vi "turning.vi"(10 "Turn time":dbl, 11 "clock anticlock":string) -> (3 "angle moved":dbl)   [LabVIEW 2015]
panel:
  out "finish angle":dbl
  out "Start angle":dbl
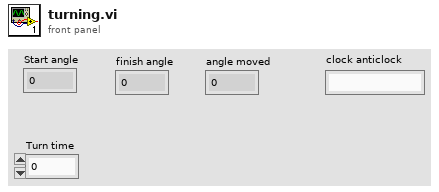
[diagram p1: front panel]
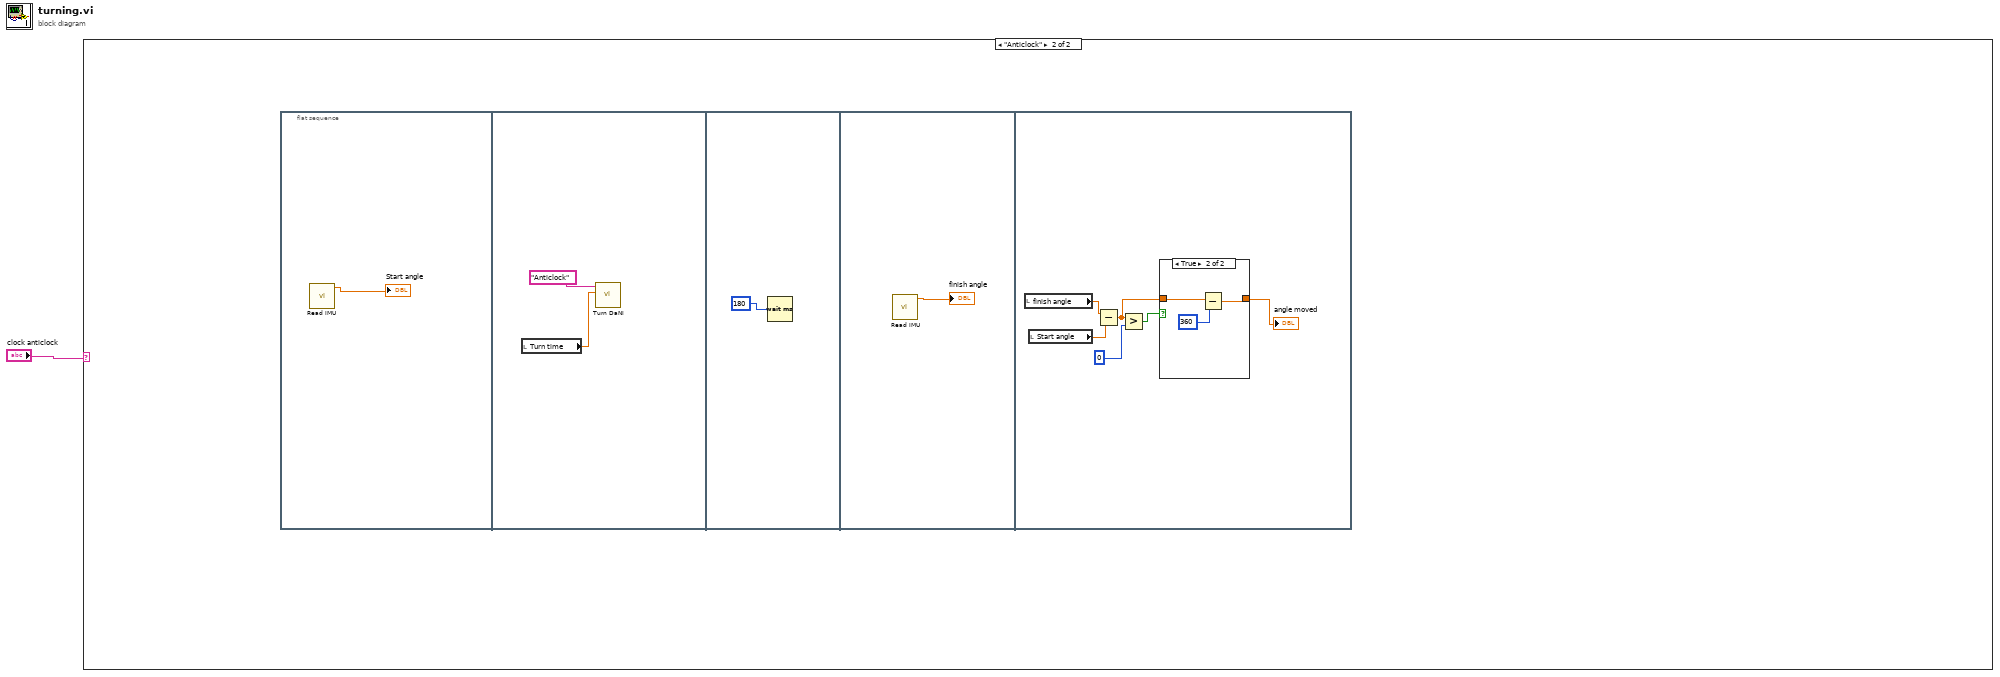
[diagram p0: block diagram]
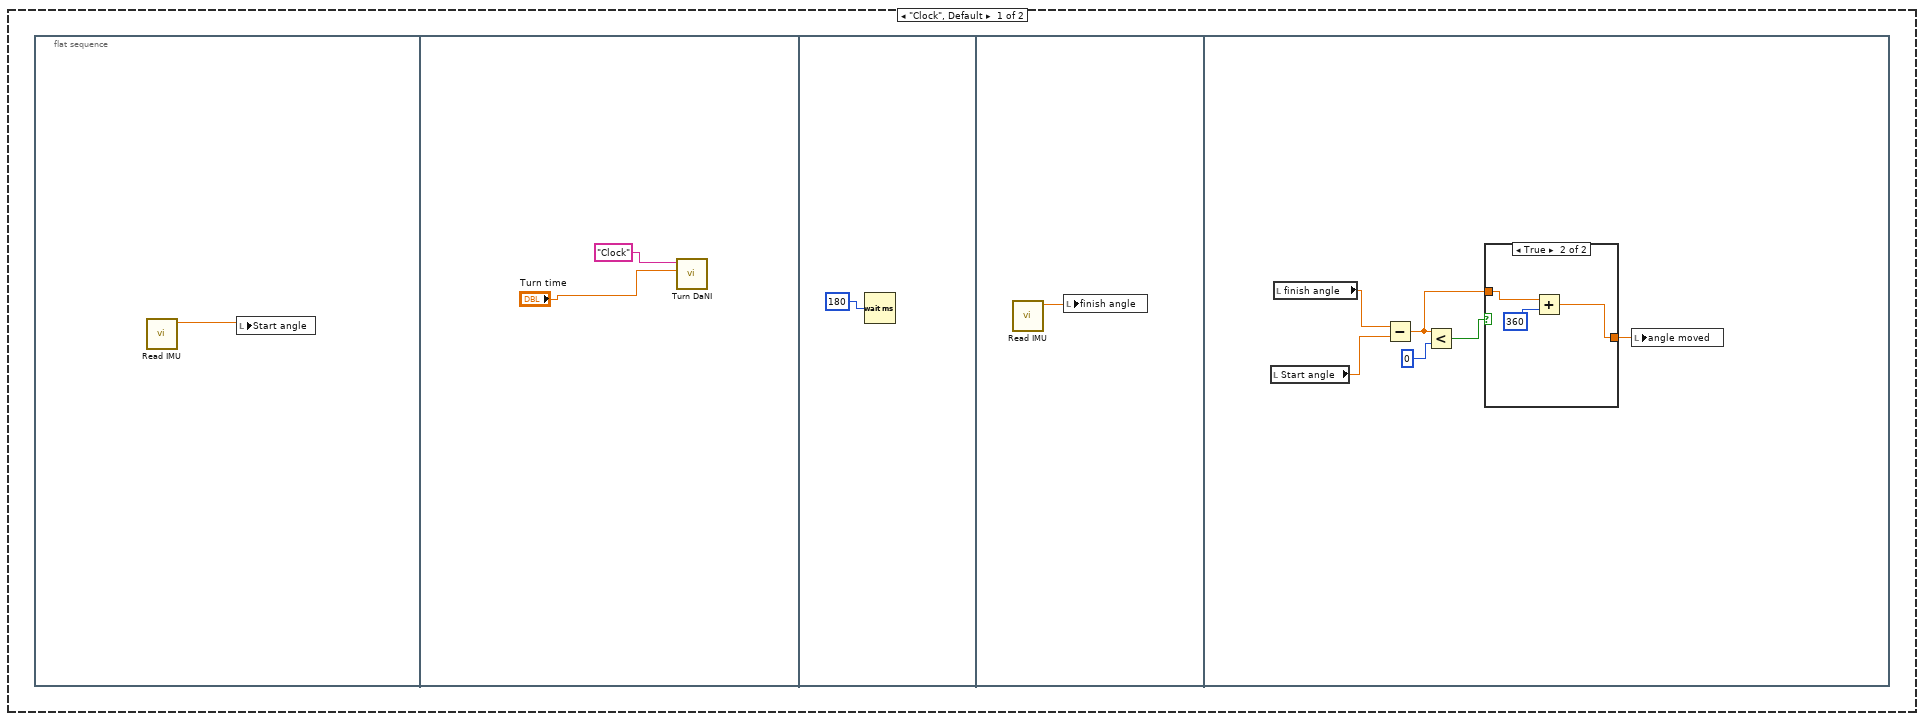
[diagram p2: hidden frame]
diagram:
  n1 = case shown="\"Anticlock\"" "clock anticlock" {
    frame "Clock", Default {
      n2 = flat-sequence {
        frame #0 {
          n3 = call "Read IMU.vi"() -> ("Output Angle"=w2:dbl)  [unwired: 10 in, 1 out]
          n4 = local write "Start angle"(w2) -> ()
        }
        frame #1 {
          n5 = call "Turn DaNI.vi"("wait time (ms)"="Turn time", "Clockwise/Anticlocwise"="Clock") -> ()  [unwired: 10 in]
        }
        frame #2 {
          n6 = Wait (ms)(milliseconds to wait=180) -> ()  [unwired: 1 out]
        }
        frame #3 {
          n7 = call "Read IMU.vi"() -> ("Output Angle"=w6:dbl)  [unwired: 10 in, 1 out]
          n8 = local write "finish angle"(w6) -> ()
        }
        frame #4 {
          n9 = local read "Start angle"() -> (w12:dbl)
          n10 = local read "finish angle"() -> (w11:dbl)
          n11 = Subtract(x=w11, y=w12) -> (x-y=w8:dbl)
          n12 = Less?(x=w8, y=0) -> (x < y?=w9:bool)
          n13 = case shown="True" w9 {
            tunnel: w8 -> [w13 w16]
            tunnel: [w13 w14] -> w7
            frame False {
            }
            frame True {
              n14 = Add(x=w16, y=360) -> (x+y=w14:dbl)
            }
          }
          n15 = local write "angle moved"(w7) -> ()
        }
      }
    }
    frame "Anticlock" {
      n16 = flat-sequence {
        frame #0 {
          n17 = call "Read IMU.vi"() -> ("Output Angle"=→"Start angle":dbl)  [unwired: 10 in, 1 out]
        }
        frame #1 {
          n18 = local read "Turn time"() -> (w18:dbl)
          n19 = call "Turn DaNI.vi"("wait time (ms)"=w18, "Clockwise/Anticlocwise"="Anticlock") -> ()  [unwired: 10 in]
        }
        frame #2 {
          n20 = Wait (ms)(milliseconds to wait=180) -> ()  [unwired: 1 out]
        }
        frame #3 {
          n21 = call "Read IMU.vi"() -> ("Output Angle"=→"finish angle":dbl)  [unwired: 10 in, 1 out]
        }
        frame #4 {
          n22 = local read "finish angle"() -> (w26:dbl)
          n23 = local read "Start angle"() -> (w27:dbl)
          n24 = Subtract(x=w26, y=w27) -> (x-y=w23:dbl)
          n25 = Greater?(x=w23, y=0) -> (0:w25:bool)
          n26 = case shown="True" w25 {
            tunnel: w23 -> [w28 w31]
            tunnel: [w28 w29] -> w22
            frame False {
            }
            frame True {
              n27 = Subtract(x=w31, y=360) -> (x-y=w29:dbl)
            }
          }
          "angle moved" <- w22
        }
      }
    }
  }
